vi "Basicincrement.vi"() -> ()   [LabVIEW 2015]
panel:
  in  "stop":bool
  out "Numeric":dbl
  in  "Boolean":bool
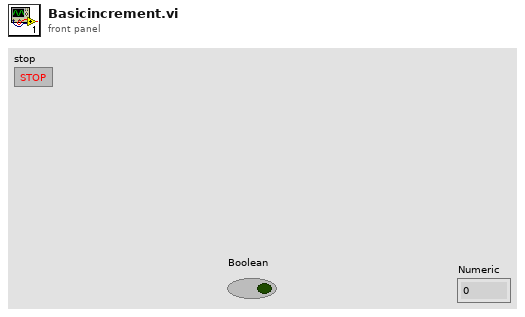
[diagram p1: front panel]
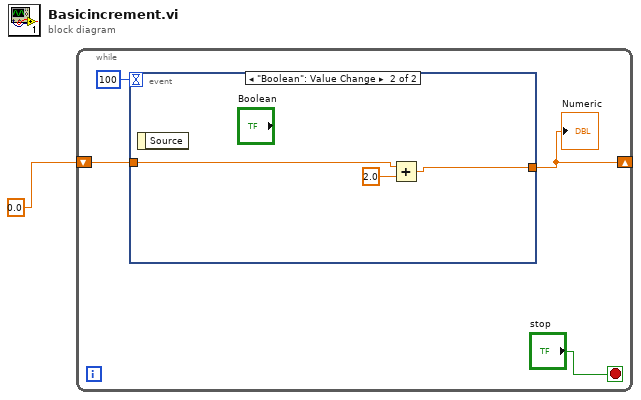
[diagram p0: block diagram]
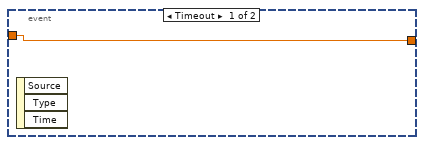
[diagram p2: hidden frame]
diagram:
  n1 = while {
    shift-right: [w2] -> _
    shift-left: 0.0 -> [w4]
    stop <- "stop" stop-if-true
    n2 = event shown="[1] \"Boolean\": Value Change" {
      selector: _ -> [_ _]
      dyn-events: _ -> [_ _]
      timeout: 100 -> [_ _]
      tunnel: w4 -> [w6 w8]
      tunnel: [w6 w7] -> w2
      event Timeout {
        n3 = event-data() -> ()  [unwired: 1 in, 3 out]
      }
      event "Boolean": Value Change {
        n4 = event-data() -> ()  [unwired: 1 in, 1 out]
        n5 = Add(x=w8, y=2.0) -> (x+y=w7:dbl)
      }
    }
    "Numeric" <- w2
  }
